vi "AO Repeat.vi"() -> ()   [LabVIEW 2019]
uses:
  <vilib>/rvi/Emulation/niFpgaGetClockAttributes.vi
  <vilib>/rvi/Emulation/niFpgaSctlEmulationGetInTimedLoop.vi
  <vilib>/rvi/Emulation/niFpgaEmulationReportErrorSimple.vi
  <vilib>/rvi/Emulation/niFpgaProcessEmulError.vi
  <vilib>/rvi/DataTransferAndStorage/Container/Common/niFpgaContainerGetUniqueNameForEmu.vi
  <vilib>/rvi/DataTransferAndStorage/Container/Common/niFpgaContainerSetEmuInfo.vi
  <vilib>/rvi/eio/common/nirviEmuReportErrorAndStop.vi
  <vilib>/rvi/DataTransferAndStorage/Container/Common/niFpgaContainerExecOnDevCompGetState.vi
  <vilib>/rvi/Emulation/niFpgaEmulationIsFPGAContextNoSignature.vi
  <vilib>/rvi/errors/nirviReportUnexpectedCaseInternalError (U32).vi
  <vilib>/rvi/Memory/Memory_Emulation/niFpgaMemoryEmulationCacheClearOnFirstRun.vi
  <vilib>/rvi/Memory/Memory_Emulation/nirvimemoryEmulationManagerCache_MakeExclusive.vi
  <vilib>/rvi/Memory/Memory_Emulation/niFpgaMemoryEmulationValidateCache.vi
  <vilib>/rvi/Memory/Memory_Emulation/nirvimemoryEmulationManagerCache_InsertValue.vi
  <vilib>/Utility/error.llb/Clear Errors.vi
  <vilib>/rvi/Memory/Memory_Emulation/nirvimemoryEmulationManagerCache_ReleaseExclusive.vi
  <vilib>/rvi/Memory/Memory_Emulation/nirvimemoryEmulationManagerCache_GetValue.vi
  <vilib>/rvi/Memory/Memory_Emulation/nirvimemoryEmulationManagerCache_SetValue.vi
  <vilib>/rvi/Emulation/niFpgaSctlEmulationResourceMgr.vi
  <vilib>/rvi/eio/common/nirviEmuTemplateMethod_errors.vi
  <vilib>/rvi/Emulation/niFpgaCriticalErrorInLSC.vi
  <vilib>/rvi/interface/RandomDataEmulation/nirviRandomDataMultiElementFPGAFIFO.vi
  <instcachedir>/0/nirviRandomDataMultiElementFPGAFIFO_1ED88BA00AC641F388A9B1FAA20E354D.lvgen/nirviRandomDataMultiElementFPGAFIFO_1ED88BA00AC641F388A9B1FAA20E354D_005.vi
  <vilib>/rvi/interface/RandomDataEmulation/niFpgaRandomDataHandleErrors.vi
  <vilib>/rvi/LocalResourceManager/LocalResourceManager.xnode
  <vilib>/rvi/DataTransferAndStorage/Container/XNode/niFpgaContainer.xnode
  <vilib>/rvi/Memory/Memory_Emulation/niFpgaMemoryEmulationRefIn.vi
  <vilib>/eio/EIONode/EIONode.xnode
  <vilib>/rvi/interface/RandomDataEmulation/nirviRandomDataFpgaMultiElementTemplate.vi
panel:
  in  "CNTRB1":u32=200
  in  "CNTRB0":u32=200
  in  "CNTRA1":u32=200
  in  "存储.数据量B1":u32
  in  "存储.数据量B0":u32
  in  "存储.数据量A1":u32
  in  "B1.Enable":bool
  in  "B0.Enable":bool
  in  "A1.Enable":bool
  in  "A0.Enable":bool
  in  "CNTRA0":u32=200
  in  "开始":bool
  in  "存储.数据量A0":u32
  in  "Reset":bool
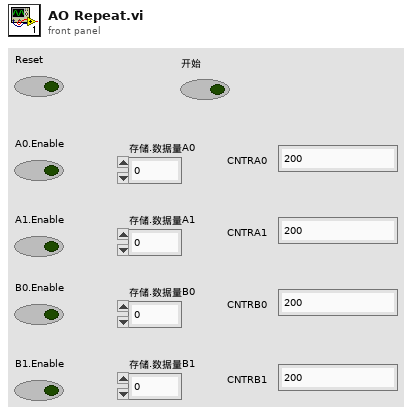
[diagram p1: front panel]
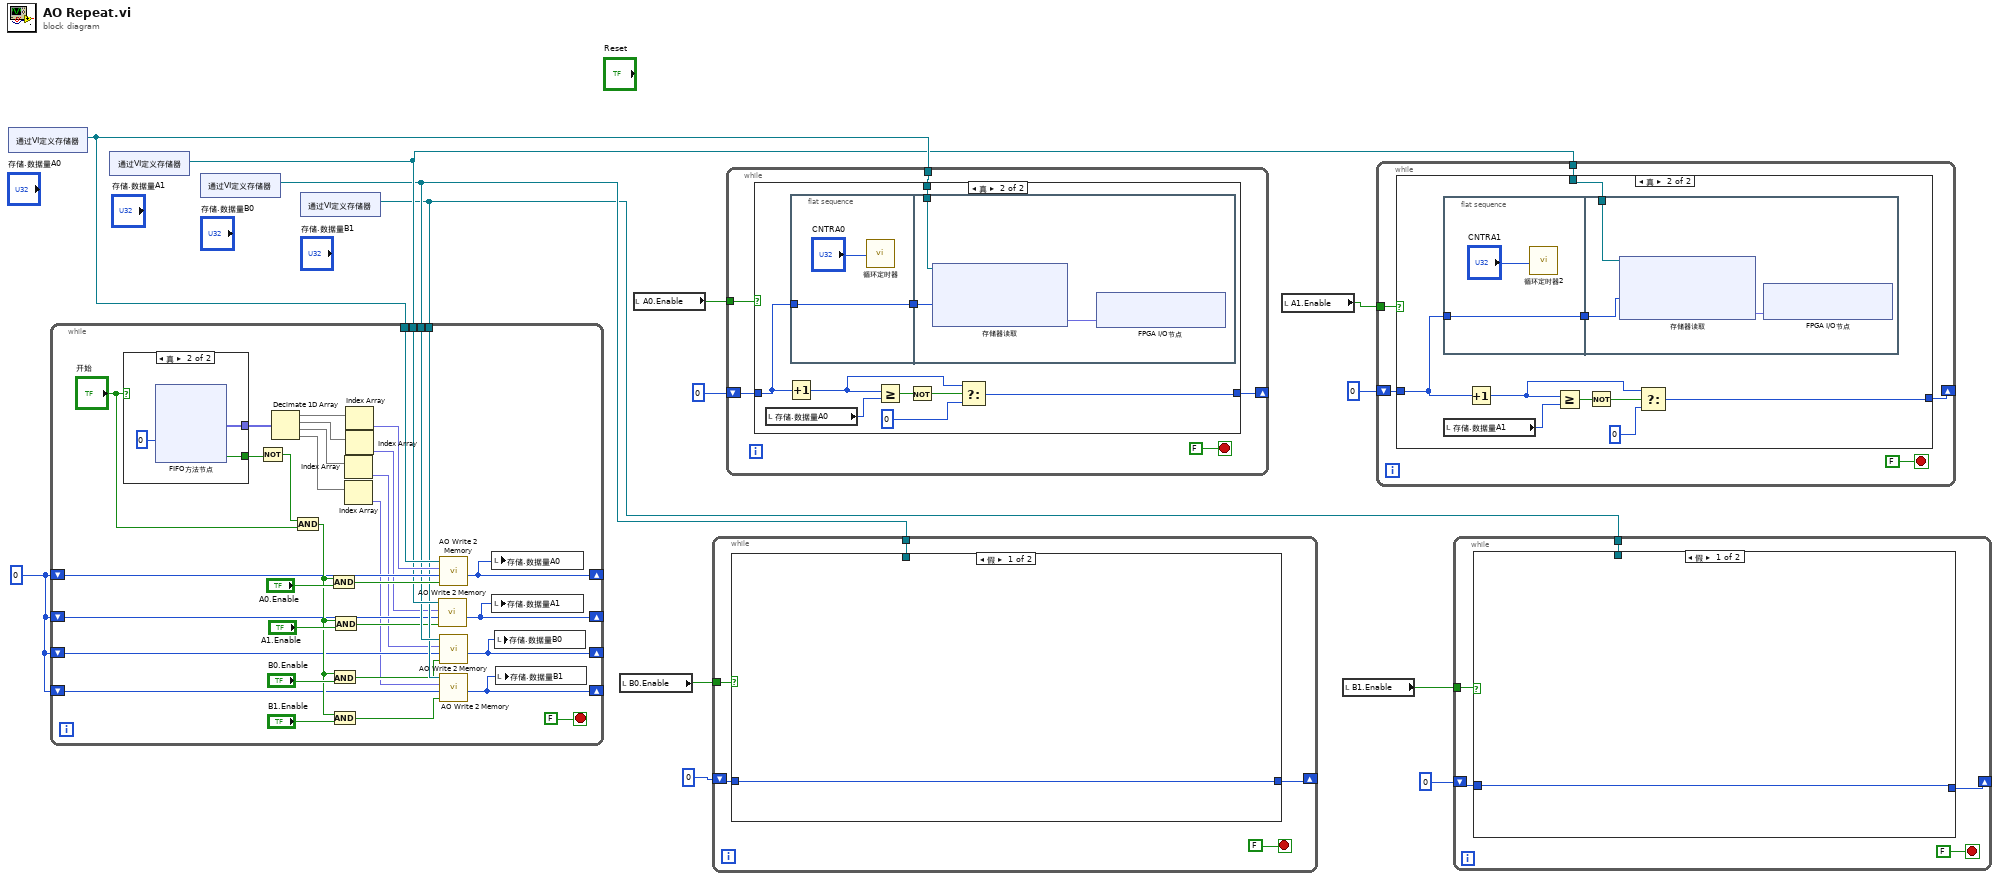
[diagram p0: block diagram]
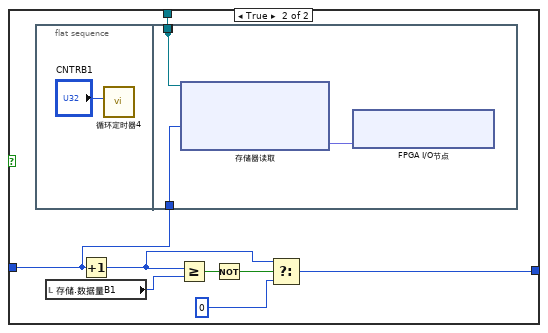
[diagram p2: hidden frame]
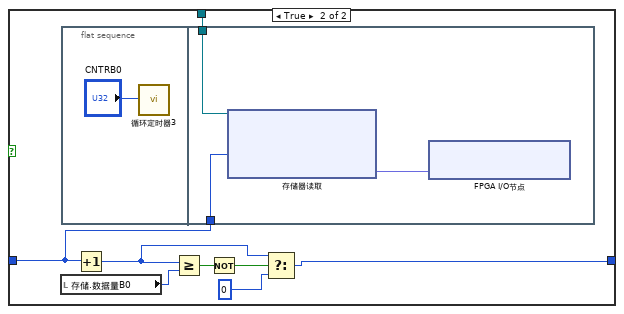
[diagram p3: hidden frame]
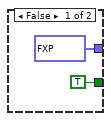
[diagram p6: hidden frame]
diagram:
  w13 = u32 0 ("存储.数据量A0")
  n1 = xnode "通过VI定义存储器"() -> ("存储器输出"=w12:refnum<k21>)
  n2 = xnode "通过VI定义存储器"() -> ("存储器输出"=w10:refnum<k21>)
  n3 = xnode "通过VI定义存储器"() -> ("存储器输出"=w9:refnum<k21>)
  n4 = xnode "通过VI定义存储器"() -> ("存储器输出"=w8:refnum<k21>)
  n5 = while {
    shift-right: [w32] -> _
    shift-left: w13 -> [w35]
    tunnel: w12 -> [w33]
    tunnel: w10 -> [w31]
    tunnel: w9 -> [w30]
    tunnel: w8 -> [w29]
    shift-right: [w16] -> _
    shift-left: w13 -> [w25]
    shift-right: [w15] -> _
    shift-left: w13 -> [w23]
    shift-right: [w14] -> _
    shift-left: w13 -> [w24]
    stop <- FALSE stop-if-true
    n6 = case shown="真" "开始" {
      tunnel: [fxp<+/-,20,5>[] [0.0, 0.0, 0.0, 0.0] ("元素") w51] -> w44
      tunnel: [TRUE ("超时？") w50] -> w47
      frame False {
      }
      frame True {
        n7 = xnode ("FIFO方法节点")("超时"=0) -> ("元素"=w51:fxp<+/-,20,5>[], "超时？"=w50:bool)  [unwired: 1 in, 1 out]
      }
    }
    n8 = Not(x=w47) -> (.not. x?=w46:bool)
    n9 = Decimate 1D Array(w44) -> (w37:fxp<+/-,20,5>[], w22:fxp<+/-,20,5>[], w21:fxp<+/-,20,5>[], w20:fxp<+/-,20,5>[])
    n10 = And(x=w46, y="开始") -> (x .and. y?=w39:bool)
    n11 = And(x=w39, y="A0.Enable") -> (x .and. y?=w34:bool)
    n12 = And(x=w39, y="B0.Enable") -> (x .and. y?=w27:bool)
    n13 = And(x=w39, y="B1.Enable") -> (x .and. y?=w26:bool)
    n14 = And(x=w39, y="A1.Enable") -> (x .and. y?=w28:bool)
    n15 = Index Array(array=w21) -> (element=w18:fxp<+/-,20,5>)  [unwired: 1 in]
    n16 = Index Array(array=w20) -> (element=w17:fxp<+/-,20,5>)  [unwired: 1 in]
    n17 = Index Array(array=w37) -> (element=w36:fxp<+/-,20,5>)  [unwired: 1 in]
    n18 = Index Array(array=w22) -> (element=w19:fxp<+/-,20,5>)  [unwired: 1 in]
    n19 = call "AO Write 2 Memory.vi"("Enable"=w28, "地址 i"=w25, "数值"=w19, "存储器输入"=w31) -> ("地址 i+1"=w16:u32)  [unwired: 7 in]
    n20 = call "AO Write 2 Memory.vi"("Enable"=w34, "地址 i"=w35, "数值"=w36, "存储器输入"=w33) -> ("地址 i+1"=w32:u32)  [unwired: 7 in]
    n21 = call "AO Write 2 Memory.vi"("Enable"=w27, "地址 i"=w23, "数值"=w18, "存储器输入"=w30) -> ("地址 i+1"=w15:u32)  [unwired: 7 in]
    n22 = call "AO Write 2 Memory.vi"("Enable"=w26, "地址 i"=w24, "数值"=w17, "存储器输入"=w29) -> ("地址 i+1"=w14:u32)  [unwired: 7 in]
    n23 = local write "存储.数据量A0"(w32) -> ()
    n24 = local write "存储.数据量A1"(w16) -> ()
    n25 = local write "存储.数据量B0"(w15) -> ()
    n26 = local write "存储.数据量B1"(w14) -> ()
  }
  n27 = local read "B0.Enable"() -> (w2:bool)
  n28 = local read "A0.Enable"() -> (w4:bool)
  n29 = while {
    tunnel: w9 -> [w57]
    shift-right: [w56] -> _
    shift-left: u32 0 ("存储.数据量A0") -> [w54]
    tunnel: w2 -> [w53]
    stop <- FALSE stop-if-true
    n30 = case shown="假" w53 {
      tunnel: w57 -> [_ w66]
      tunnel: [w58 w62] -> w56
      tunnel: w54 -> [w58 w60]
      frame False {
      }
      frame True {
        n31 = local read "存储.数据量B0"() -> (w61:u32)
        n32 = flat-sequence {
          tunnel: w66 -> [w70]
          tunnel: w60 -> [w69]
          frame #0 {
            n33 = call "循环定时器3"("Count(Ticks)"="CNTRB0") -> ()  [unwired: 1 out]
          }
          frame #1 {
            n34 = xnode "存储器读取"("地址"=w69, "存储器输入"=w70) -> ("数据"=w68:fxp<+/-,20,5>)  [unwired: 1 out]
            n35 = xnode "FPGA I/O节点"("ConnectorB/AO0"=w68) -> ()  [unwired: 1 in, 1 out]
          }
        }
        n36 = Increment(x=w60) -> (x+1=w63:u32)
        n37 = Greater Or Equal?(x=w63, y=w61) -> (x >= y?=w65:bool)
        n38 = Not(x=w65) -> (.not. x?=w64:bool)
        n39 = Select(t=w63, s=w64, f=u32 0 ("存储.数据量A0")) -> (s? t:f=w62:u32)
      }
    }
  }
  n40 = while {
    tunnel: w12 -> [w73]
    shift-right: [w74] -> _
    shift-left: u32 0 ("存储.数据量A0") -> [w75]
    tunnel: w4 -> [w71]
    stop <- FALSE stop-if-true
    n41 = case shown="真" w71 {
      tunnel: w75 -> [w76 w83]
      tunnel: [w76 w78] -> w74
      tunnel: w73 -> [_ w77]
      frame False {
      }
      frame True {
        n42 = local read "存储.数据量A0"() -> (w84:u32)
        n43 = Increment(x=w83) -> (x+1=w79:u32)
        n44 = flat-sequence {
          tunnel: [w86] -> w85
          tunnel: w83 -> [w86]
          tunnel: w85 -> [w89]
          tunnel: w77 -> [w90]
          frame #0 {
            n45 = call "循环定时器"("Count(Ticks)"="CNTRA0") -> ()  [unwired: 1 out]
          }
          frame #1 {
            n46 = xnode "存储器读取"("地址"=w89, "存储器输入"=w90) -> ("数据"=w88:fxp<+/-,20,5>)  [unwired: 1 out]
            n47 = xnode "FPGA I/O节点"("ConnectorA/AO0"=w88) -> ()  [unwired: 1 in, 1 out]
          }
        }
        n48 = Greater Or Equal?(x=w79, y=w84) -> (x >= y?=w82:bool)
        n49 = Not(x=w82) -> (.not. x?=w81:bool)
        n50 = Select(t=w79, s=w81, f=u32 0 ("存储.数据量A0")) -> (s? t:f=w78:u32)
      }
    }
  }
  n51 = local read "A1.Enable"() -> (w3:bool)
  n52 = local read "B1.Enable"() -> (w1:bool)
  n53 = while {
    tunnel: w10 -> [w92]
    shift-right: [w95] -> _
    shift-left: u32 0 ("存储.数据量A0") -> [w93]
    tunnel: w3 -> [w91]
    stop <- FALSE stop-if-true
    n54 = case shown="真" w91 {
      tunnel: [w96 w101] -> w95
      tunnel: w93 -> [w96 w99]
      tunnel: w92 -> [_ w98]
      frame False {
      }
      frame True {
        n55 = flat-sequence {
          tunnel: [w106] -> w105
          tunnel: w99 -> [w106]
          tunnel: w105 -> [w109]
          tunnel: w98 -> [w110]
          frame #0 {
            n56 = call "循环定时器2"("Count(Ticks)"="CNTRA1") -> ()  [unwired: 1 out]
          }
          frame #1 {
            n57 = xnode "存储器读取"("地址"=w109, "存储器输入"=w110) -> ("数据"=w108:fxp<+/-,20,5>)  [unwired: 1 out]
            n58 = xnode "FPGA I/O节点"("ConnectorA/AO1"=w108) -> ()  [unwired: 1 in, 1 out]
          }
        }
        n59 = local read "存储.数据量A1"() -> (w100:u32)
        n60 = Increment(x=w99) -> (x+1=w102:u32)
        n61 = Greater Or Equal?(x=w102, y=w100) -> (x >= y?=w104:bool)
        n62 = Not(x=w104) -> (.not. x?=w103:bool)
        n63 = Select(t=w102, s=w103, f=u32 0 ("存储.数据量A0")) -> (s? t:f=w101:u32)
      }
    }
  }
  n64 = while {
    tunnel: w8 -> [w115]
    shift-right: [w114] -> _
    shift-left: u32 0 ("存储.数据量A0") -> [w112]
    tunnel: w1 -> [w111]
    stop <- FALSE stop-if-true
    n65 = case shown="假" w111 {
      tunnel: w115 -> [_ w124]
      tunnel: [w116 w120] -> w114
      tunnel: w112 -> [w116 w118]
      frame False {
      }
      frame True {
        n66 = flat-sequence {
          tunnel: [w128] -> _
          tunnel: w124 -> [w128]
          tunnel: w118 -> [w127]
          frame #0 {
            n67 = call "循环定时器4"("Count(Ticks)"="CNTRB1") -> ()  [unwired: 1 out]
          }
          frame #1 {
            n68 = xnode "存储器读取"("地址"=w127, "存储器输入"=w128) -> ("数据"=w126:fxp<+/-,20,5>)  [unwired: 1 out]
            n69 = xnode "FPGA I/O节点"("ConnectorB/AO1"=w126) -> ()  [unwired: 1 in, 1 out]
          }
        }
        n70 = local read "存储.数据量B1"() -> (w119:u32)
        n71 = Increment(x=w118) -> (x+1=w121:u32)
        n72 = Greater Or Equal?(x=w121, y=w119) -> (x >= y?=w123:bool)
        n73 = Not(x=w123) -> (.not. x?=w122:bool)
        n74 = Select(t=w121, s=w122, f=u32 0 ("存储.数据量A0")) -> (s? t:f=w120:u32)
      }
    }
  }
